vi "OutputErrorPoly.vi"   [LabVIEW 2013]
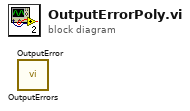
[diagram p0: block diagram]
diagram:
  n1 = call "OutputErrors.vi"() -> ()  [unwired: 11 in, 1 out]
  n2 = call "OutputError.vi"() -> ()  [unwired: 11 in, 1 out]
